vi "BatchRead.vi"(5 "点数":i16=10 min=1 max=960 step=1, 7 "软元件":string="D0", 8 "错误输入":errorcluster caption="错误输入（无错误）", 11 "连接":T1={"目的端口"=65502, "网络地址"=0, "连接ID"=refnum}) -> (0 "错误输出":errorcluster, 1 "输出数组":u16[](array[numeric])=[1234, 12592, 0, 19328, 0, 0, 27380, 824, 28836, 16709] format="%04x", 2 "时间":dbl=3611280816.8313456 format="%#.6f秒", 3 "连接ID 2":refnum<k16>, 4 "数据输出":string)   [LabVIEW 2018]
panel:
  out "连接的字符串":string
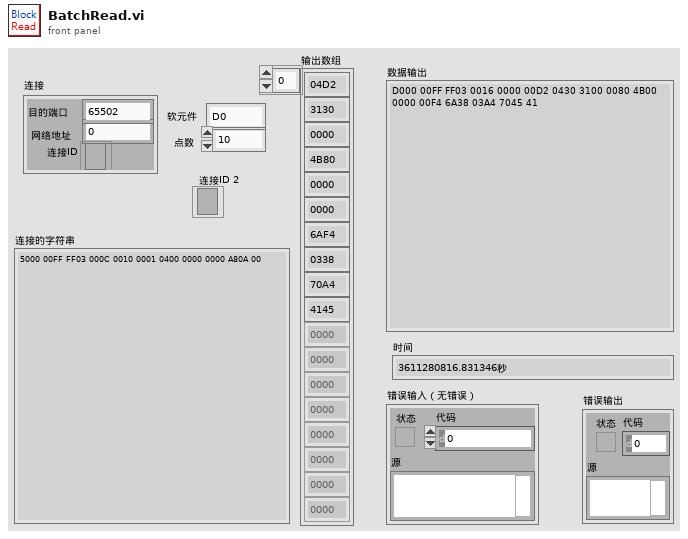
[diagram p1: front panel]
types:
  T1 = cluster{"目的端口":u16, "网络地址":u32, "连接ID":refnum<k16>}
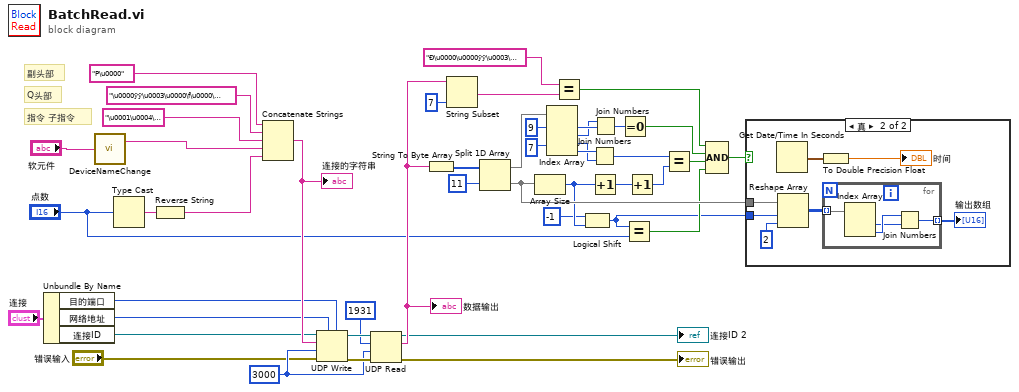
[diagram p0: block diagram]
diagram:
  w36 = 3000 ("超时毫秒(25000)")
  # "指令 子指令"
  # "Q头部"
  # "副头部"
  n1 = Unbundle By Name("连接") -> ("目的端口"=w2:u16, "网络地址"=w1:u32, "连接ID"=w3:refnum<k16>)
  n2 = call "DeviceNameChange.vi"("软元件"="软元件") -> ("字符串"=w43:string)  [unwired: 1 out]
  n3 = Type Cast(x="点数") -> (*(type *) &x=w45:string)  [unwired: 1 in]
  n4 = Reverse String(1:w45) -> (0:w44:string)
  n5 = Concatenate Strings("P\u0000", "\u0000ÿÿ\u0003\u0000\f\u0000\u0010\u0000", "\u0001\u0004\u0000\u0000", w43, w44) -> (w39:string)
  "连接的字符串" <- w39
  n6 = UDP Write(address=w1, port or service name=w2, connection ID=w3, data in=w39, 8:"错误输入", 9:w36) -> (error out=w37:errorcluster, 3:w38:refnum<k16>)
  n7 = UDP Read(connection ID=w38, max size (548)=1931 ("最大值(548)"), timeout ms (25000)=w36, 8:w37) -> (data out=w31:string, error out=→"错误输出":errorcluster, 3:→"连接ID 2":refnum<k16>)  [unwired: 2 out]
  "数据输出" <- w31
  n8 = String To Byte Array(string=w31) -> (unsigned byte array=w34:u8[])
  n9 = String Subset(string=w31, length (rest)=7 ("长度（剩余）")) -> (substring=w28:string)  [unwired: 1 in]
  n10 = Split 1D Array(array=w34, index=11 ("索引")) -> (first subarray=w32:u8[], second subarray=w16:u8[])
  n11 = Array Size(array=w16) -> (size(s)=w12:i32)
  n12 = Index Array(array=w32, index #1=9 ("索引"), index #3=7 ("索引")) -> (element #1=w24:u8, element #2=w23:u8, element #3=w25:u8, element #4=w26:u8)  [unwired: 2 in]
  n13 = Equal?(x="Ð\u0000\u0000ÿÿ\u0003\u0000", y=w28) -> (x = y?=w13:bool)
  n14 = Logical Shift ("逻辑移位")(y=i8 -1, x=w12) -> (x << y=w8:i32)
  n15 = Join Numbers(hi=w26, lo=w25) -> ((hi.lo)=w18:u16)
  n16 = Increment(x=w12) -> (x+1=w22:i32)
  n17 = Join Numbers(hi=w23, lo=w24) -> ((hi.lo)=w20:u16)
  n18 = Equal To 0?(x=w20) -> (x = 0?=w14:bool)
  n19 = Equal?(x=w8, y="点数") -> (x = y?=w10:bool)
  n20 = Increment(x=w22) -> (x+1=w19:i32)
  n21 = Equal?(x=w18, y=w19) -> (x = y?=w15:bool)
  n22 = Compound Arithmetic op=AND(w13, w14, w15, w10) -> (w17:bool)
  n23 = case shown="真" w17 {
    tunnel: w16 -> [_ w53]
    tunnel: w8 -> [_ w52]
    frame False {
    }
    frame True {
      n24 = Get Date/Time In Seconds() -> (seconds since 1Jan1904=w48:timestamp)
      n25 = Reshape Array ("重排数组维数")(w53, w52, 2 ("维数大小")) -> (w50:u8[][])
      n26 = To Double Precision Float(number=w48) -> (double precision float=→"时间":dbl)
      n27 = for {
        tunnel: w50 -> [w57] mode=indexing
        tunnel: [w54] -> w49 mode=indexing
        n28 = Index Array(array=w57) -> (element #1=w55:u8, element #2=w56:u8)  [unwired: 2 in]
        n29 = Join Numbers(hi=w56, lo=w55) -> ((hi.lo)=w54:u16)
      }
      "输出数组" <- w49
    }
  }
